vi "对中 转动角度判断.vi"() -> ()   [LabVIEW 2015, in "Logging.lvlib"]
uses:
  Logging.lvlib
panel:
  out "转动？":bool
  in  "对称性合格条件":dbl
  in  "扭矩对称轴":dbl
  in  "对称性":dbl
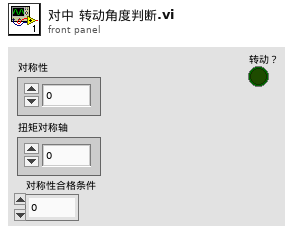
[diagram p1: front panel]
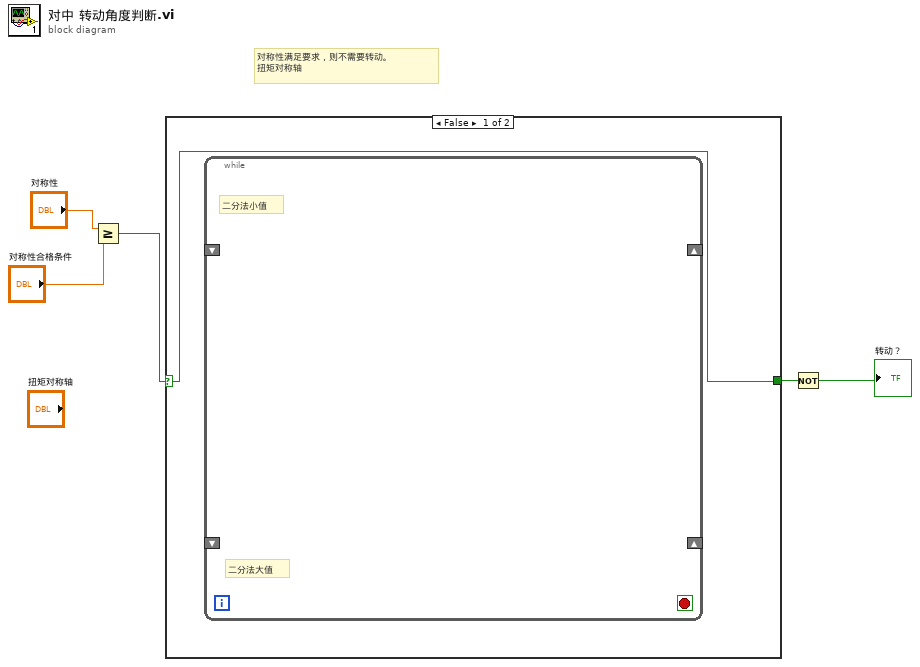
[diagram p0: block diagram]
diagram:
  # "对称性满足要求，则不需要转动。\n扭矩对称轴"
  n1 = Greater Or Equal?(x="对称性", y="对称性合格条件") -> (x >= y?=w3:bool)
  n2 = case shown="False" w3 {
    selector: w3 -> [w6 w7]
    tunnel: [w6 w7] -> w2
    frame False {
      n3 = while {
        shift-right: _ -> [_]
        shift-left: _ -> [_]
        shift-right: _ -> [_]
        shift-left: _ -> [_]
        stop <- _ stop-if-true
        # "二分法大值"
        # "二分法小值"
      }
    }
    frame True {
    }
  }
  n4 = Not(x=w2) -> (.not. x?=→"转动？":bool)
